vi "standard_cmd_write.vi"(5 "COM":bool, 6 "error in (no error)":errorcluster, 7 "VISA name":refnum<visa-resource-name>, 8 "data":u8[](array[numeric]), 9 "dwLen":u32, 10 "dwAddr":u32, 11 "cmd_std_header_t":T1) -> (3 "return":i32, 4 "error out":errorcluster)   [LabVIEW 2016]
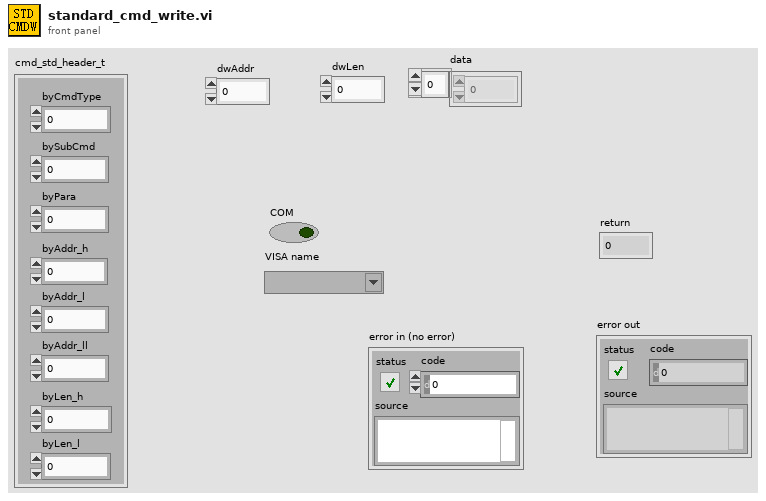
[diagram p1: front panel]
types:
  T1 = cluster{"byCmdType":u8, "bySubCmd":u8, "byPara":u8, "byAddr_h":u8, "byAddr_l":u8, "byAddr_ll":u8, "byLen_h":u8, "byLen_l":u8}
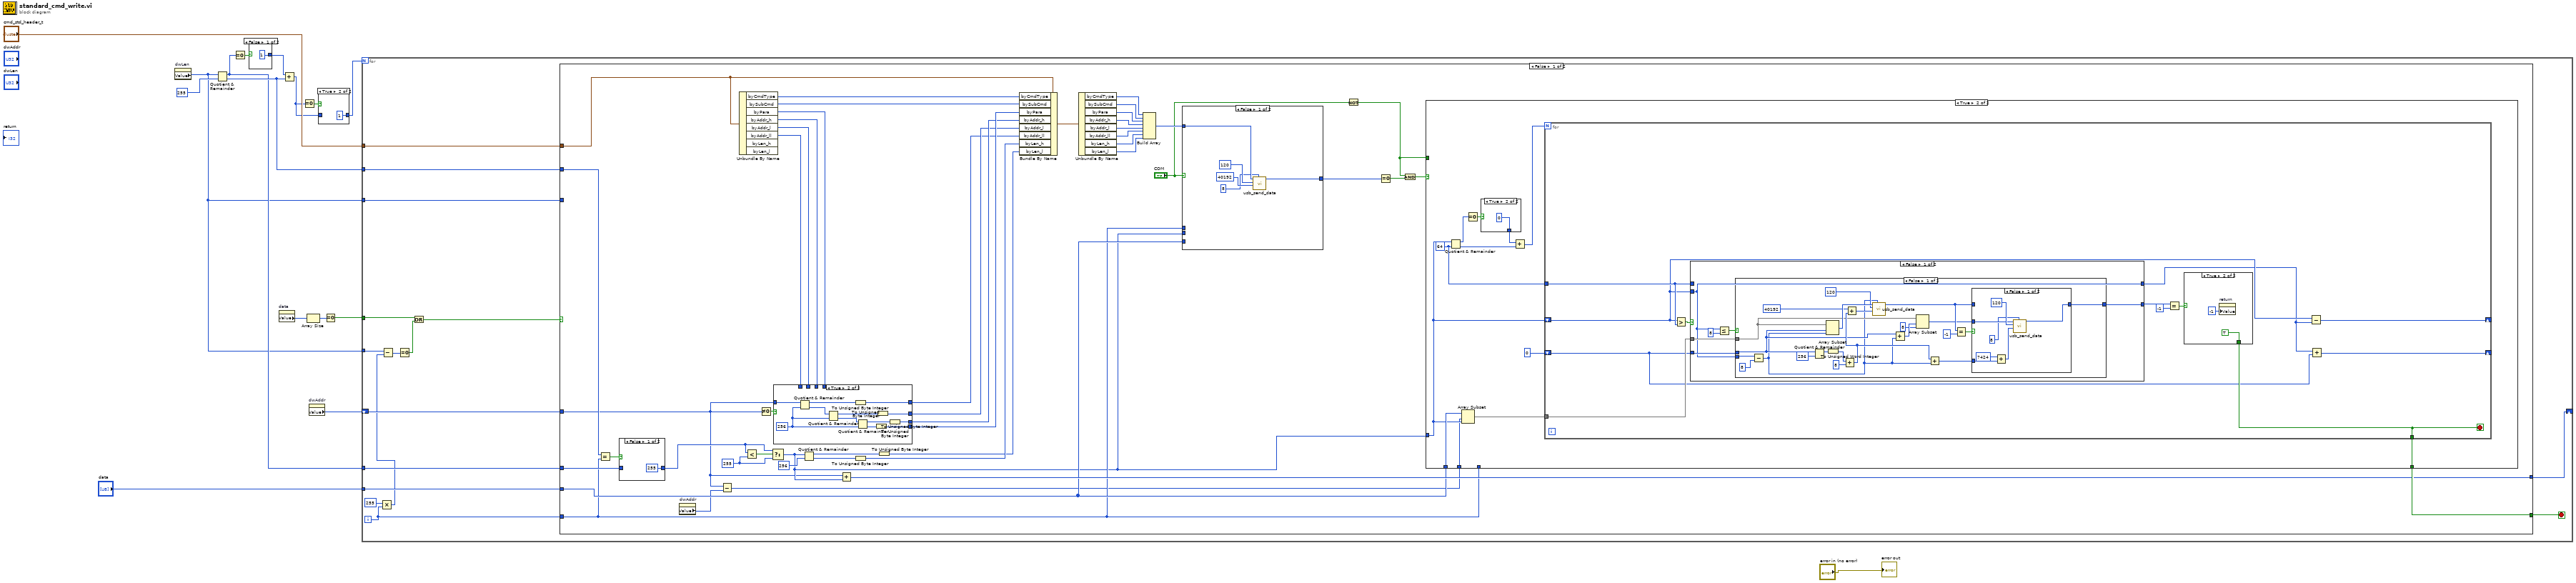
[diagram p0: block diagram]
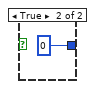
[diagram p3: hidden frame]
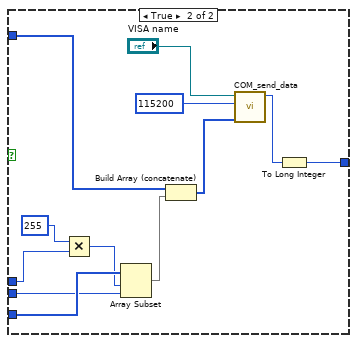
[diagram p4: hidden frame]
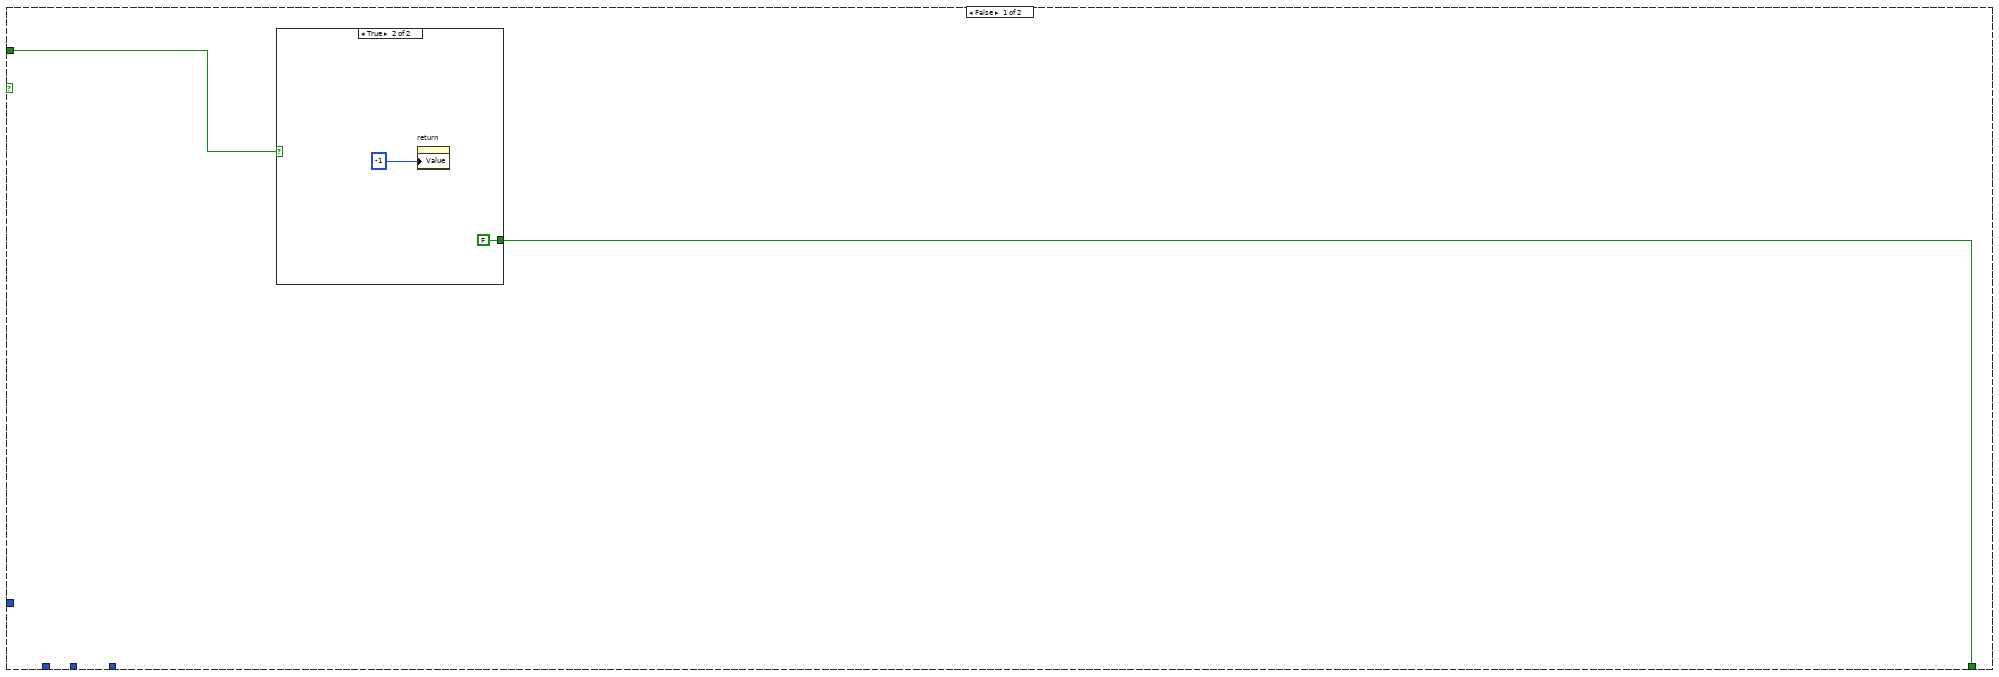
[diagram p6: hidden frame]
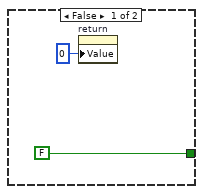
[diagram p7: hidden frame]
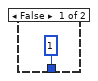
[diagram p8: hidden frame]
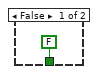
[diagram p9: hidden frame]
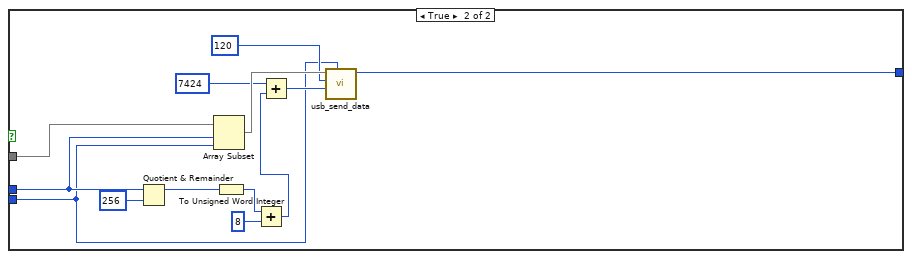
[diagram p11: hidden frame]
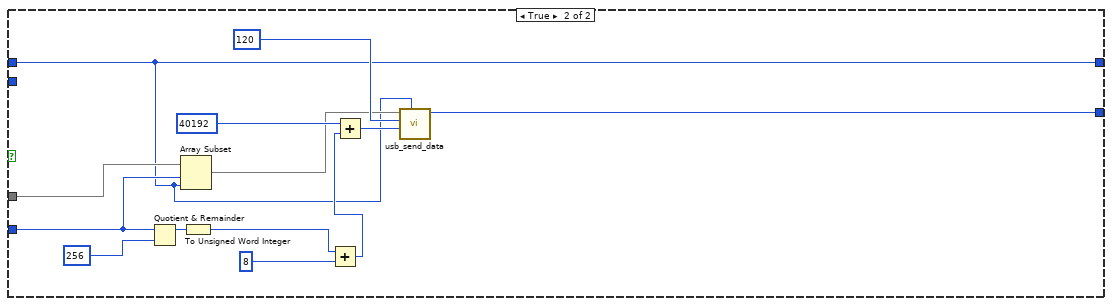
[diagram p12: hidden frame]
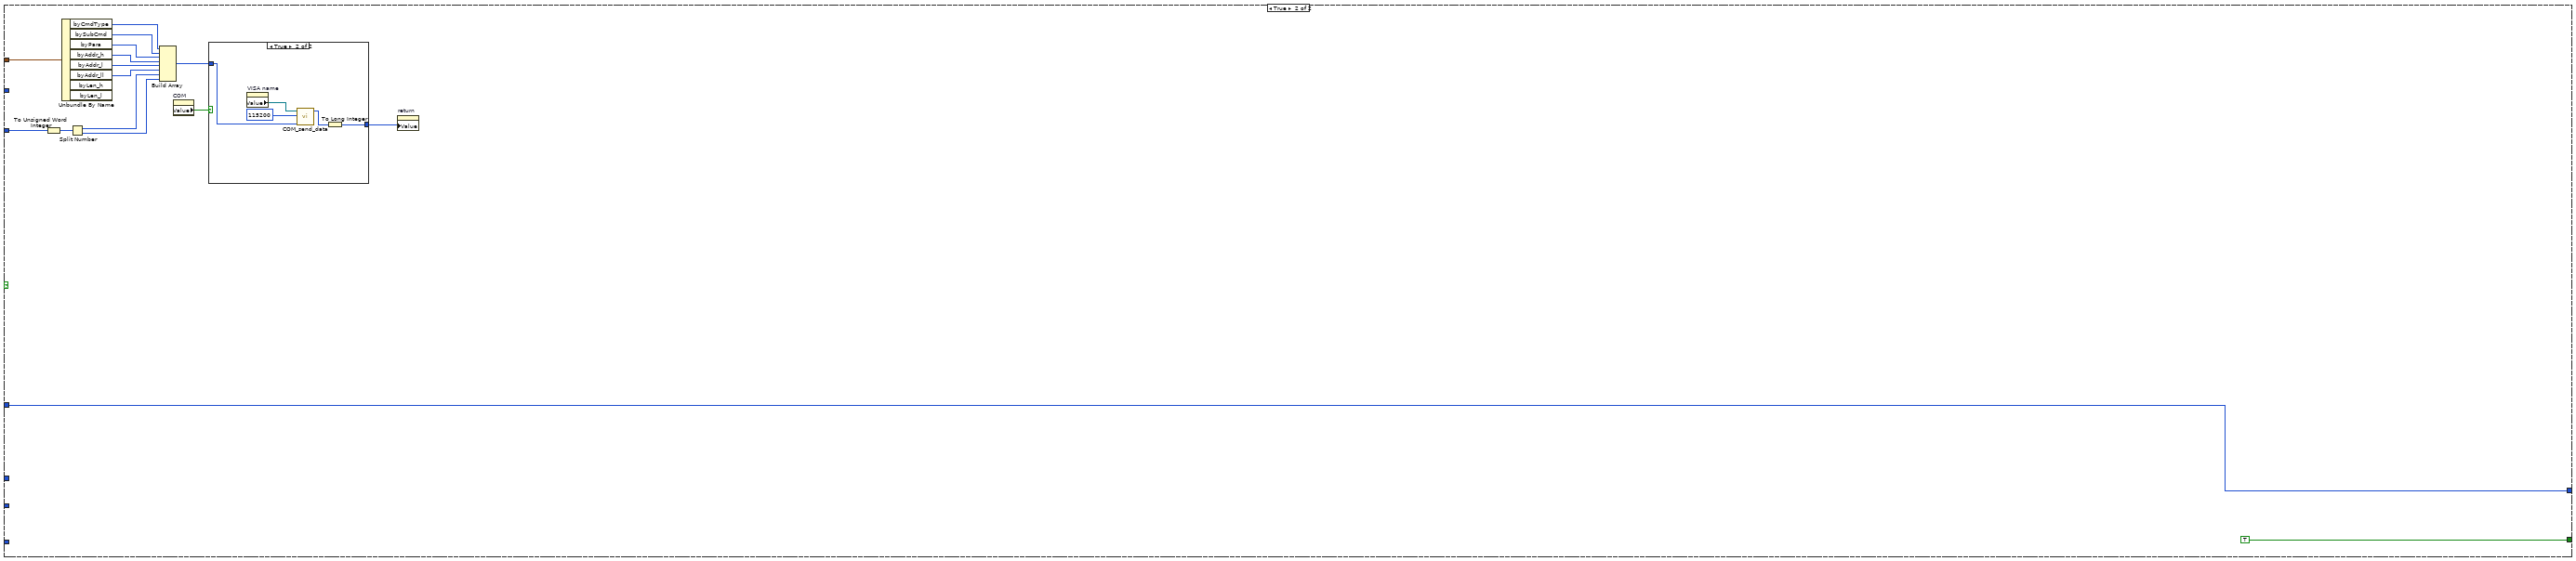
[diagram p14: hidden frame]
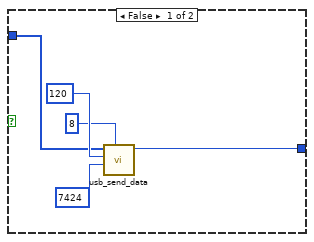
[diagram p15: hidden frame]
diagram:
  n1 = property on="dwLen" class="DigNum (strict)"() -> ("Value"=w2:u32)  [unwired: 2 in, 2 out]
  n2 = Quotient & Remainder(x=w2, y=u32 255) -> (x-y*floor(x/y)=w11:u32, floor(x/y)=w12:u32)
  n3 = Equal To 0?(x=w11) -> (x = 0?=w14:bool)
  n4 = case shown="False" w14 {
    tunnel: [u32 1 u32 0] -> w13
    frame False {
    }
    frame True {
    }
  }
  n5 = property on="data" class="Arr (strict)"() -> ("Value"=w8:u8[])  [unwired: 2 in, 2 out]
  n6 = Add(x=w13, y=w12) -> (x+y=w4:u32)
  n7 = Equal To 0?(x=w4) -> (x = 0?=w5:bool)
  n8 = Array Size(array=w8) -> (size(s)=w7:i32)
  n9 = property on="dwAddr" class="DigNum (strict)"() -> ("Value"=w9:u32)  [unwired: 2 in, 2 out]
  n10 = case shown="True" w5 {
    tunnel: w4 -> [w19 _]
    tunnel: [w19 u32 1] -> w3
    frame False {
    }
    frame True {
    }
  }
  n11 = Equal To 0?(x=w7) -> (x = 0?=w6:bool)
  n12 = for {
    N: w3 -> [_]
    tunnel: "cmd_std_header_t" -> [w36]
    tunnel: w12 -> [w34]
    tunnel: w11 -> [w33]
    shift-right: [w31] -> _
    shift-left: w9 -> [w32]
    tunnel: w2 -> [w29]
    tunnel: w6 -> [w23]
    tunnel: "data" -> [w30]
    tunnel: w2 -> [w21]
    i -> [w28]
    stop <- w35 stop-if-true
    n13 = Multiply(x=255, y=w28) -> (x*y=w26:i32)
    n14 = Subtract(x=w29, y=w26) -> (x-y=w25:u32)
    n15 = Equal To 0?(x=w25) -> (x = 0?=w24:bool)
    n16 = Or(x=w23, y=w24) -> (x .or. y?=w22:bool)
    n17 = case shown="False" w22 {
      tunnel: w36 -> [w79 w229]
      tunnel: [w63 TRUE] -> w35
      tunnel: w34 -> [w61 _]
      tunnel: w33 -> [w60 _]
      tunnel: w32 -> [w39 w221]
      tunnel: [w58 w221] -> w31
      tunnel: w30 -> [w46 _]
      tunnel: w28 -> [w45 _]
      tunnel: w21 -> [_ w217]
      frame False {
        w81 = u32 255 ("f")
        n18 = Equal?(x=w61, y=w45) -> (x = y?=w62:bool)
        n19 = case shown="False" w62 {
          tunnel: w60 -> [_ w101]
          tunnel: [u32 255 w101] -> w59
          frame False {
          }
          frame True {
          }
        }
        n20 = property on="dwAddr" class="DigNum (strict)"() -> ("Value"=w38:u32)  [unwired: 2 in, 2 out]
        n21 = Subtract(x=w39, y=w38) -> (x-y=w37:u32)
        n22 = Unbundle By Name(w79) -> ("byCmdType"=w65:u8, "bySubCmd"=w64:u8, "byPara"=w69:u8, "byAddr_h"=w68:u8, "byAddr_l"=w67:u8, "byAddr_ll"=w66:u8)  [unwired: 2 out]
        n23 = Less?(x=w59, y=w81) -> (x < y?=w82:bool)
        n24 = Not Equal To 0?(x=w39) -> (x != 0?=w70:bool)
        n25 = Select(t=w59, s=w82, f=w81) -> (s? t:f=w44:u32)
        n26 = case shown="True" w70 {
          tunnel: w39 -> [_ w214]
          tunnel: [w202 w209] -> w78
          tunnel: [w201 w205] -> w73
          tunnel: [w200 w204] -> w72
          tunnel: [w199 w203] -> w71
          tunnel: w69 -> [w202 _]
          tunnel: w68 -> [w201 _]
          tunnel: w67 -> [w200 _]
          tunnel: w66 -> [w199 _]
          frame False {
          }
          frame True {
            w211 = u32 256 ("y")
            n27 = Quotient & Remainder(x=w214, y=w211) -> (x-y*floor(x/y)=w206:u32, floor(x/y)=w213:u32)
            n28 = Quotient & Remainder(x=w213, y=w211) -> (x-y*floor(x/y)=w207:u32, floor(x/y)=w212:u32)
            n29 = To Unsigned Byte Integer(number=w206) -> (unsigned 8bit integer=w203:u8)
            n30 = Quotient & Remainder(x=w212, y=w211) -> (x-y*floor(x/y)=w208:u32, floor(x/y)=w210:u32)
            n31 = To Unsigned Byte Integer(number=w210) -> (unsigned 8bit integer=w209:u8)
            n32 = To Unsigned Byte Integer(number=w207) -> (unsigned 8bit integer=w204:u8)
            n33 = To Unsigned Byte Integer(number=w208) -> (unsigned 8bit integer=w205:u8)
          }
        }
        n34 = Quotient & Remainder(x=w44, y=u32 256) -> (x-y*floor(x/y)=w76:u32, floor(x/y)=w77:u32)
        n35 = Add(x=w39, y=w44) -> (x+y=w58:u32)
        n36 = To Unsigned Byte Integer(number=w77) -> (unsigned 8bit integer=w75:u8)
        n37 = To Unsigned Byte Integer(number=w76) -> (unsigned 8bit integer=w74:u8)
        n38 = Bundle By Name(cluster=w79, "byCmdType"=w65, "bySubCmd"=w64, "byPara"=w78, "byAddr_h"=w73, "byAddr_l"=w72, "byAddr_ll"=w71, "byLen_h"=w75, "byLen_l"=w74) -> (w56:T1)
        n39 = Unbundle By Name(w56) -> ("byCmdType"=w55:u8, "bySubCmd"=w54:u8, "byPara"=w53:u8, "byAddr_h"=w52:u8, "byAddr_l"=w51:u8, "byAddr_ll"=w50:u8, "byLen_h"=w49:u8, "byLen_l"=w48:u8)
        n40 = Build Array(w55, w54, w53, w52, w51, w50, w49, w48) -> (w47:u8[])
        n41 = case shown="False" "COM" {
          tunnel: [w85 w88] -> w57
          tunnel: w47 -> [w84 w92]
          tunnel: w46 -> [_ w97]
          tunnel: w45 -> [_ w95]
          tunnel: w44 -> [_ w96]
          frame False {
            n42 = call "usb_send_data.vi"("byVdCmdHeaderLen"=u16 8, "I2C_VD_BUFFER_RW"=u16 40192, "I2C_SLAVE_ID"=u8 120, "data"=w84) -> ("return"=w85:i32)  [unwired: 6 in, 1 out]
          }
          frame True {
            n43 = Multiply(x=255, y=w95) -> (x*y=w93:i32)
            n44 = Array Subset(array=w97, index=w93, length=w96) -> (w91:u8[])
            n45 = Build Array (concatenate)(w92, w91) -> (w90:u8[])
            n46 = call "COM_send_data.vi"("data"=w90, "baud rate (9600)"=u32 115200, "VISA name"="VISA name") -> ("return"=w89:i32)  [unwired: 8 in]
            n47 = To Long Integer(number=w89) -> (32bit integer=w88:i32)
          }
        }
        n48 = Not(x="COM") -> (.not. x?=w40:bool)
        n49 = Equal To 0?(x=w57) -> (x = 0?=w41:bool)
        n50 = And(x=w40, y=w41) -> (x .and. y?=w43:bool)
        n51 = case shown="True" w43 {
          tunnel: [w102 w112] -> w63
          tunnel: w44 -> [_ w110]
          tunnel: w46 -> [_ w111]
          tunnel: w45 -> [_ _]
          tunnel: w40 -> [w103 _]
          tunnel: w37 -> [_ w109]
          frame False {
            n52 = case shown="True" w103 {
              tunnel: [FALSE FALSE] -> w102
              frame False {
                n53 = property on="return" class="DigNum (strict)"("Value"=0 ("return")) -> ()  [unwired: 2 in, 2 out]
              }
              frame True {
                n54 = property on="return" class="DigNum (strict)"("Value"=-1 ("return")) -> ()  [unwired: 2 in, 2 out]
              }
            }
          }
          frame True {
            w114 = u32 64 ("y")
            n55 = Quotient & Remainder(x=w110, y=w114) -> (x-y*floor(x/y)=w118:u32, floor(x/y)=w116:u32)
            n56 = Array Subset(array=w111, index=w109, length=w110) -> (w108:u8[])
            n57 = Equal To 0?(x=w118) -> (x = 0?=w119:bool)
            n58 = case shown="True" w119 {
              tunnel: [u32 1 ("x-y*floor(x/y)") u32 0 ("x-y*floor(x/y)")] -> w117
              frame False {
              }
              frame True {
              }
            }
            n59 = Add(x=w117, y=w116) -> (x+y=w115:u32)
            n60 = for {
              N: w115 -> [_]
              shift-right: [w122] -> _
              shift-left: w110 -> [w126]
              tunnel: w114 -> [w132]
              shift-right: [w123] -> _
              shift-left: u32 0 -> [w124]
              tunnel: w108 -> [w131]
              tunnel: [w127] -> w112
              stop <- w127 stop-if-true
              n61 = Greater?(x=w126, y=w132) -> (0:w133:bool)
              n62 = case shown="False" w133 {
                tunnel: w132 -> [_ w186]
                tunnel: w126 -> [w138 _]
                tunnel: [w138 w186] -> w125
                tunnel: w124 -> [w141 w189]
                tunnel: w131 -> [w140 w191]
                tunnel: [w142 w187] -> w129
                frame False {
                  n63 = Less Or Equal?(x=w138, y=u32 8) -> (x <= y?=w139:bool)
                  n64 = case shown="False" w139 {
                    tunnel: [w153 w177] -> w142
                    tunnel: w141 -> [w149 w176]
                    tunnel: w140 -> [w146 w175]
                    tunnel: w138 -> [w157 w173]
                    frame False {
                      n65 = Subtract(x=w157, y=u32 8) -> (x-y=w143:u32)
                      n66 = Quotient & Remainder(x=w149, y=u32 256) -> (x-y*floor(x/y)=w163:u32)  [unwired: 1 out]
                      n67 = Array Subset(array=w146, index=w149, length=w143) -> (w161:u8[])
                      n68 = To Unsigned Word Integer(number=w163) -> (unsigned 16bit integer=w162:u16)
                      n69 = Add(x=w162, y=u16 8) -> (x+y=w151:u16)
                      n70 = Add(x=u16 40192 ("I2C_VD_BUFFER_RW"), y=w151) -> (x+y=w164:u16)
                      n71 = call "usb_send_data.vi"("byVdCmdHeaderLen"=w143, "I2C_VD_BUFFER_RW"=w164, "I2C_SLAVE_ID"=u8 120, "data"=w161) -> ("return"=w152:i32)  [unwired: 6 in, 1 out]
                      n72 = Add(x=w149, y=w143) -> (x+y=w148:u32)
                      n73 = Array Subset(array=w146, index=w148, length=8) -> (w145:u8[])
                      n74 = Add(x=w151, y=w143) -> (x+y=w150:u32)
                      n75 = Equal?(x=w152, y=-1) -> (x = y?=w155:bool)
                      n76 = case shown="False" w155 {
                        tunnel: [w171 w172] -> w153
                        tunnel: w152 -> [_ w172]
                        tunnel: w150 -> [w170 _]
                        tunnel: w145 -> [w166 _]
                        frame False {
                          n77 = Add(x=u32 7424, y=w170) -> (x+y=w169:u32)
                          n78 = call "usb_send_data.vi"("byVdCmdHeaderLen"=u16 8, "I2C_VD_BUFFER_RW"=w169, "I2C_SLAVE_ID"=u8 120, "data"=w166) -> ("return"=w171:i32)  [unwired: 6 in, 1 out]
                        }
                        frame True {
                        }
                      }
                    }
                    frame True {
                      n79 = Quotient & Remainder(x=w176, y=u32 256) -> (x-y*floor(x/y)=w184:u32)  [unwired: 1 out]
                      n80 = Array Subset(array=w175, index=w176, length=w173) -> (w181:u8[])
                      n81 = To Unsigned Word Integer(number=w184) -> (unsigned 16bit integer=w183:u16)
                      n82 = Add(x=w183, y=u16 8) -> (x+y=w182:u16)
                      n83 = Add(x=u16 7424 ("I2C_VD_BUFFER_RW"), y=w182) -> (x+y=w185:u16)
                      n84 = call "usb_send_data.vi"("byVdCmdHeaderLen"=w173, "I2C_VD_BUFFER_RW"=w185, "I2C_SLAVE_ID"=u8 120, "data"=w181) -> ("return"=w177:i32)  [unwired: 6 in, 1 out]
                    }
                  }
                }
                frame True {
                  n85 = Quotient & Remainder(x=w189, y=u32 256) -> (x-y*floor(x/y)=w195:u32)  [unwired: 1 out]
                  n86 = Array Subset(array=w191, index=w189, length=w186) -> (w188:u8[])
                  n87 = To Unsigned Word Integer(number=w195) -> (unsigned 16bit integer=w194:u16)
                  n88 = Add(x=w194, y=u16 8) -> (x+y=w192:u16)
                  n89 = Add(x=u16 40192 ("I2C_VD_BUFFER_RW"), y=w192) -> (x+y=w197:u16)
                  n90 = call "usb_send_data.vi"("byVdCmdHeaderLen"=w186, "I2C_VD_BUFFER_RW"=w197, "I2C_SLAVE_ID"=u8 120, "data"=w188) -> ("return"=w187:i32)  [unwired: 6 in, 1 out]
                }
              }
              n91 = Equal?(x=w129, y=-1) -> (x = y?=w130:bool)
              n92 = case shown="True" w130 {
                tunnel: [FALSE TRUE] -> w127
                frame False {
                }
                frame True {
                  n93 = property on="return" class="DigNum (strict)"("Value"=-1 ("return")) -> ()  [unwired: 2 in, 2 out]
                }
              }
              n94 = Subtract(x=w126, y=w125) -> (x-y=w122:u32)
              n95 = Add(x=w125, y=w124) -> (x+y=w123:u32)
            }
          }
        }
      }
      frame True {
        n96 = To Unsigned Word Integer(number=w217) -> (unsigned 16bit integer=w218:u16)
        n97 = Unbundle By Name(w229) -> ("byCmdType"=w228:u8, "bySubCmd"=w227:u8, "byPara"=w226:u8, "byAddr_h"=w225:u8, "byAddr_l"=w224:u8, "byAddr_ll"=w223:u8)  [unwired: 2 out]
        n98 = Split Number(x=w218) -> (hi(x)=w216:u8, lo(x)=w215:u8)
        n99 = Build Array(w228, w227, w226, w225, w224, w223, w216, w215) -> (w222:u8[])
        n100 = property on="COM" class="Bool (strict)"() -> ("Value"=w220:bool)  [unwired: 2 in, 2 out]
        n101 = case shown="True" w220 {
          tunnel: w222 -> [w233 w238]
          tunnel: [w232 w236] -> w219
          frame False {
            n102 = call "usb_send_data.vi"("byVdCmdHeaderLen"=u16 8, "I2C_VD_BUFFER_RW"=u16 7424, "I2C_SLAVE_ID"=u8 120, "data"=w233) -> ("return"=w232:i32)  [unwired: 6 in, 1 out]
          }
          frame True {
            n103 = property on="VISA name" class="VISAName"() -> ("Value"=w240:refnum<visa-resource-name>)  [unwired: 2 in, 2 out]
            n104 = call "COM_send_data.vi"("data"=w238, "baud rate (9600)"=u32 115200, "VISA name"=w240) -> ("return"=w237:i32)  [unwired: 8 in]
            n105 = To Long Integer(number=w237) -> (32bit integer=w236:i32)
          }
        }
        n106 = property on="return" class="DigNum (strict)"("Value"=w219) -> ()  [unwired: 2 in, 2 out]
      }
    }
  }
  "error out" <- "error in (no error)"
